vi "json_word.vi"(5 "text":string, 7 "ch":string, 9 "at":i32, 11 "error in (no error)":errorcluster) -> (4 "word":variant, 8 "ch out":string, 10 "at out":i32, 15 "error out":errorcluster)   [LabVIEW 2011]
doc: "Parse a \"true\", \"false\", or \"null\" value. Nulls are returned as empty variants. (Not perfect, but LV doesn't have anything like null...)"
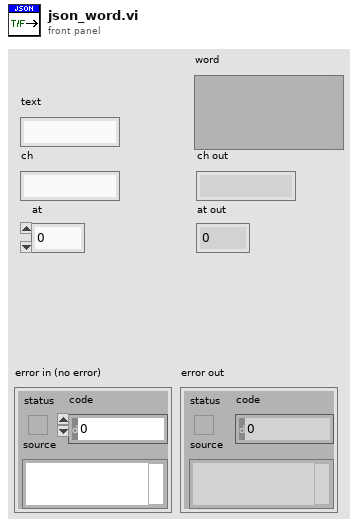
[diagram p1: front panel]
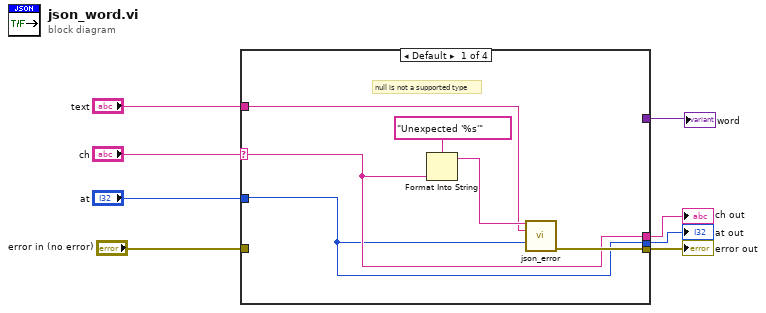
[diagram p0: block diagram]
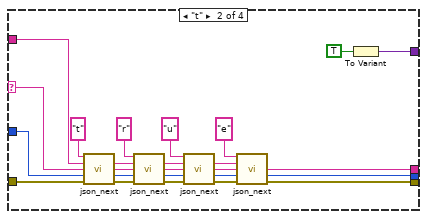
[diagram p2: hidden frame]
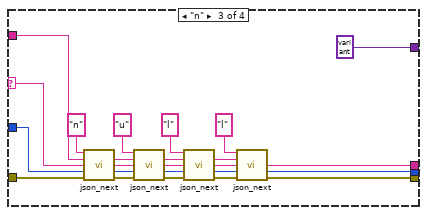
[diagram p3: hidden frame]
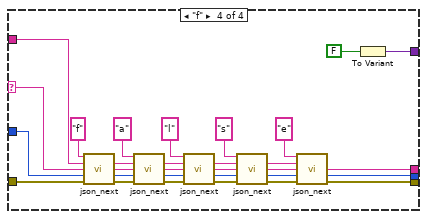
[diagram p4: hidden frame]
diagram:
  n1 = case shown="Default" "ch" {
    selector: "ch" -> [w10 w37 w61 w90]
    tunnel: "error in (no error)" -> [_ w39 w63 w92]
    tunnel: [w14 w32 w56 w71] -> w6
    tunnel: "text" -> [w11 w38 w62 w91]
    tunnel: "at" -> [w9 w36 w60 w89]
    tunnel: [_ w15 variant ("Variant") w64] -> w3
    tunnel: [w9 w18 w42 w67] -> w2
    tunnel: [w10 w17 w41 w66] -> w1
    frame Default {
      # "null is not a supported type"
      n2 = Format Into String(format string="Unexpected '%s'", w10) -> (resulting string=w12:string)  [unwired: 2 in, 1 out]
      n3 = call "json_error.vi"("m"=w12, "text"=w11, "at"=w9) -> ("error out"=w14:errorcluster)  [unwired: 12 in]
    }
    frame "t" {
      n4 = call "json_next.vi"("c"="t", "text"=w38, "ch"=w37, "at"=w36, "error in (no error)"=w39) -> ("text dup"=w31:string, "ch out"=w30:string, "at out"=w29:i32, "error out"=w35:errorcluster)  [unwired: 7 in]
      n5 = call "json_next.vi"("c"="r", "text"=w31, "ch"=w30, "at"=w29, "error in (no error)"=w35) -> ("text dup"=w24:string, "ch out"=w23:string, "at out"=w28:i32, "error out"=w34:errorcluster)  [unwired: 7 in]
      n6 = call "json_next.vi"("c"="u", "text"=w24, "ch"=w23, "at"=w28, "error in (no error)"=w34) -> ("text dup"=w25:string, "ch out"=w26:string, "at out"=w27:i32, "error out"=w33:errorcluster)  [unwired: 7 in]
      n7 = call "json_next.vi"("c"="e", "text"=w25, "ch"=w26, "at"=w27, "error in (no error)"=w33) -> ("ch out"=w17:string, "at out"=w18:i32, "error out"=w32:errorcluster)  [unwired: 7 in, 1 out]
      n8 = To Variant(anything=TRUE) -> (Variant=w15:variant)
    }
    frame "n" {
      n9 = call "json_next.vi"("c"="n", "text"=w62, "ch"=w61, "at"=w60, "error in (no error)"=w63) -> ("text dup"=w55:string, "ch out"=w54:string, "at out"=w53:i32, "error out"=w59:errorcluster)  [unwired: 7 in]
      n10 = call "json_next.vi"("c"="u", "text"=w55, "ch"=w54, "at"=w53, "error in (no error)"=w59) -> ("text dup"=w48:string, "ch out"=w47:string, "at out"=w52:i32, "error out"=w58:errorcluster)  [unwired: 7 in]
      n11 = call "json_next.vi"("c"="l", "text"=w48, "ch"=w47, "at"=w52, "error in (no error)"=w58) -> ("text dup"=w49:string, "ch out"=w50:string, "at out"=w51:i32, "error out"=w57:errorcluster)  [unwired: 7 in]
      n12 = call "json_next.vi"("c"="l", "text"=w49, "ch"=w50, "at"=w51, "error in (no error)"=w57) -> ("ch out"=w41:string, "at out"=w42:i32, "error out"=w56:errorcluster)  [unwired: 7 in, 1 out]
    }
    frame "f" {
      n13 = call "json_next.vi"("c"="f", "text"=w91, "ch"=w90, "at"=w89, "error in (no error)"=w92) -> ("text dup"=w85:string, "ch out"=w84:string, "at out"=w83:i32, "error out"=w88:errorcluster)  [unwired: 7 in]
      n14 = call "json_next.vi"("c"="a", "text"=w85, "ch"=w84, "at"=w83, "error in (no error)"=w88) -> ("text dup"=w78:string, "ch out"=w77:string, "at out"=w82:i32, "error out"=w87:errorcluster)  [unwired: 7 in]
      n15 = call "json_next.vi"("c"="l", "text"=w78, "ch"=w77, "at"=w82, "error in (no error)"=w87) -> ("text dup"=w79:string, "ch out"=w80:string, "at out"=w81:i32, "error out"=w86:errorcluster)  [unwired: 7 in]
      n16 = call "json_next.vi"("c"="s", "text"=w79, "ch"=w80, "at"=w81, "error in (no error)"=w86) -> ("text dup"=w68:string, "ch out"=w69:string, "at out"=w70:i32, "error out"=w71:errorcluster)  [unwired: 7 in]
      n17 = call "json_next.vi"("c"="e", "text"=w68, "ch"=w69, "at"=w70, "error in (no error)"=w71) -> ("ch out"=w66:string, "at out"=w67:i32)  [unwired: 7 in, 2 out]
      n18 = To Variant(anything=FALSE) -> (Variant=w64:variant)
    }
  }
  "error out" <- w6
  "word" <- w3
  "ch out" <- w1
  "at out" <- w2
